vi "_Limit Switch Test.vi"() -> ()   [LabVIEW 2025, in "USB IO.lvlib" / "USB IO.lvclass"]
uses:
  USB IO.lvclass
  USB-6000/USB-6000.lvclass
  USB IO.lvclass/USB IO.ctl
panel:
  out "error out 2":errorcluster
  out "error out":errorcluster
  out "Waveform Chart":dbl(graph)
  in  "stop":bool
  out "Boolean":bool
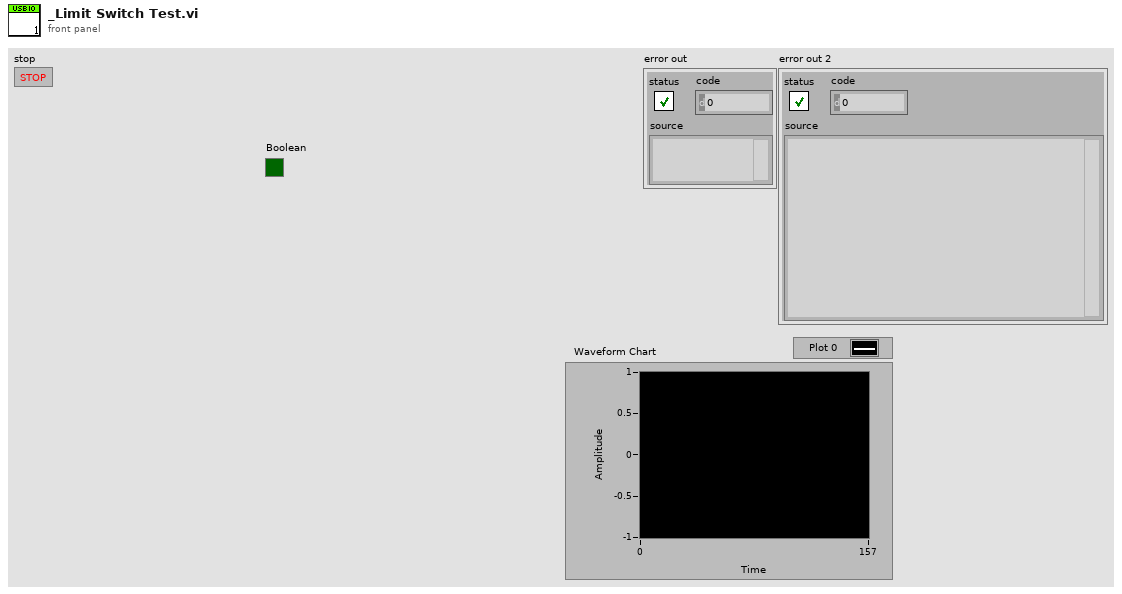
[diagram p1: front panel]
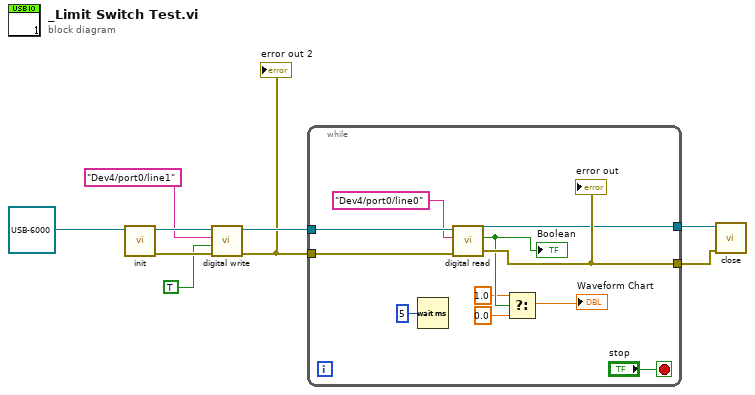
[diagram p0: block diagram]
diagram:
  n1 = call-dynamic "init.vi"("USB-6000 in"=refnum<class "USB-6000.lvclass"> refnum ("USB IO.lvlib:USB-6000.lvclass")) -> ("error out"=w6:errorcluster, "USB-6000 out"=w8:refnum<class "USB-6000.lvclass">)  [unwired: 9 in]
  n2 = call-dynamic "digital write.vi"("error in (no error)"=w6, "On/Off"=TRUE, "Line"="Dev4/port0/line1", "USB-6000 in"=w8) -> ("error out"=w3:errorcluster, "USB-6000 out"=w4:refnum<class "USB-6000.lvclass">)  [unwired: 6 in]
  "error out 2" <- w3
  n3 = while {
    tunnel: w4 -> [w20]
    tunnel: w3 -> [w19]
    tunnel: [w17] -> w2
    tunnel: [w16] -> w1
    stop <- "stop" stop-if-true
    n4 = Wait (ms)(milliseconds to wait=u32 5) -> ()  [unwired: 1 out]
    n5 = call-dynamic "digital read.vi"("error in (no error)"=w19, "Line"="Dev4/port0/line0", "USB-6000 in"=w20) -> ("error out"=w17:errorcluster, "High/Low"=w14:bool, "USB-6000 out"=w16:refnum<class "USB-6000.lvclass">)  [unwired: 6 in]
    "Boolean" <- w14
    "error out" <- w17
    n6 = Select(t=1.0, s=w14, f=0.0) -> (s? t:f=→"Waveform Chart":dbl)
  }
  n7 = call-dynamic "close.vi"("error in (no error)"=w2, "USB-6000 in"=w1) -> ()  [unwired: 8 in, 2 out]
